vi "waveformTimeKeep.vi"(4 "t0":timestamp, 6 "DAQ Settings":T2={"RH/T Sensor VSS (V)"=5.048, "K0"=0.9054, "K1"=-2.995, "Offset"=0.0, "Gain"=1.0, "Samples/Channel/s"=1000.0, "Samples to Average"=100.0} {"Offset" step=0.01 format="%_3f"; "K1" format="%#_13g"; "K0" format="%#_13g"; "RH/T Sensor VSS (V)" format="%.3g"}, 8 "error in (no error)":errorcluster, 11 "Cluster":T1) -> (0 "error out":errorcluster, 2 "Samples/second":dbl, 3 "appended array":waveform(dbl)[](array[waveform]))   [LabVIEW 2019, in "DAQ.lvclass"]
uses:
  DAQ.lvclass
  typeDefs/Parameters.ctl
  typeDefs/Graph.ctl
  <vilib>/Analysis/baseanly.llb/Mean (DBL).vi
  <vilib>/Analysis/NI_AALBase.lvlib
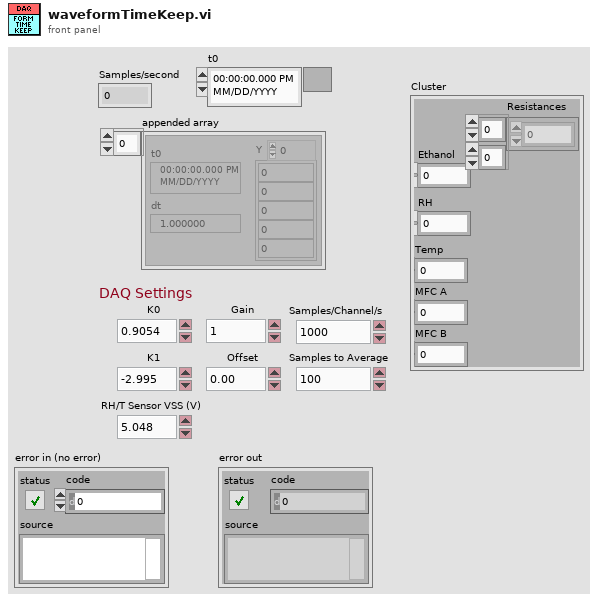
[diagram p1: front panel]
types:
  T1 = typedef "Graph.ctl" = cluster{"Ethanol":dbl, "RH":dbl, "Temp":dbl, "MFC A":dbl, "MFC B":dbl, "Resistances":dbl[][]}
  T2 = typedef "Parameters.ctl" = cluster{"RH/T Sensor VSS (V)":dbl, "K0":dbl, "K1":dbl, "Offset":dbl, "Gain":dbl, "Samples/Channel/s":dbl, "Samples to Average":dbl}
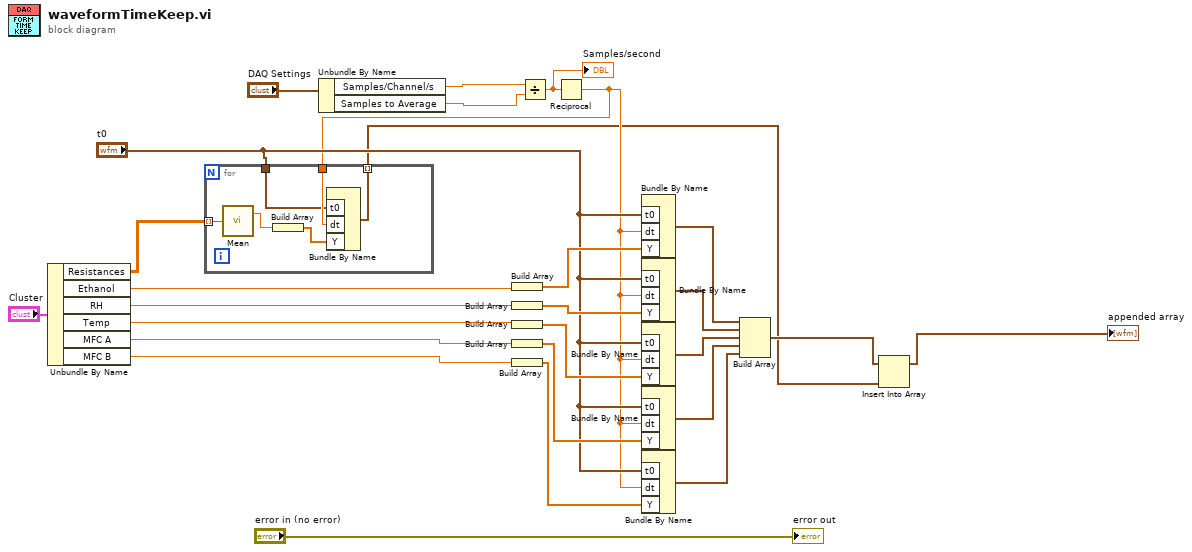
[diagram p0: block diagram]
diagram:
  n1 = Unbundle By Name("Cluster") -> ("Resistances"=w6:dbl[][], "Ethanol"=w26:dbl, "RH"=w24:dbl, "Temp"=w22:dbl, "MFC A"=w20:dbl, "MFC B"=w18:dbl)
  n2 = Unbundle By Name("DAQ Settings") -> ("Samples/Channel/s"=w9:dbl, "Samples to Average"=w10:dbl)
  n3 = Build Array(w26) -> (w25:dbl[])
  n4 = Build Array(w24) -> (w23:dbl[])
  n5 = Build Array(w22) -> (w21:dbl[])
  n6 = Build Array(w20) -> (w19:dbl[])
  n7 = Build Array(w18) -> (w17:dbl[])
  n8 = Divide(x=w9, y=w10) -> (x/y=w8:dbl)
  "Samples/second" <- w8
  n9 = Reciprocal(x=w8) -> (1/x=w4:dbl)
  n10 = for {
    tunnel: w6 -> [w33] mode=indexing
    tunnel: "t0" -> [w31]
    tunnel: w4 -> [w32]
    tunnel: [w28] -> w2 mode=indexing
    n11 = call-poly <vilib>:"Mean.vi"("X"=w33) -> ("mean"=w30:dbl)  [unwired: 1 out]
    n12 = Build Array(w30) -> (w29:dbl[])
    n13 = Bundle By Name("t0"=w31, "dt"=w32, "Y"=w29) -> (w28:waveform(dbl))  [unwired: 1 in]
  }
  n14 = Bundle By Name("t0"="t0", "dt"=w4, "Y"=w25) -> (w16:waveform(dbl))  [unwired: 1 in]
  n15 = Bundle By Name("t0"="t0", "dt"=w4, "Y"=w23) -> (w15:waveform(dbl))  [unwired: 1 in]
  n16 = Bundle By Name("t0"="t0", "dt"=w4, "Y"=w21) -> (w14:waveform(dbl))  [unwired: 1 in]
  n17 = Bundle By Name("t0"="t0", "dt"=w4, "Y"=w19) -> (w13:waveform(dbl))  [unwired: 1 in]
  n18 = Bundle By Name("t0"="t0", "dt"=w4, "Y"=w17) -> (w12:waveform(dbl))  [unwired: 1 in]
  n19 = Build Array(w16, w15, w14, w13, w12) -> (w3:waveform(dbl)[])
  n20 = Insert Into Array(array=w3, new element=w2) -> (→"appended array":waveform(dbl)[])  [unwired: 1 in]
  "error out" <- "error in (no error)"
